vi "create stack file name.vi"(8 "error in (no error)":errorcluster, 10 "name or relative path":string, 11 "Autofocus in":refnum<class "Autofocus.lvclass">) -> (0 "error out":errorcluster, 1 "stack base_xy":path, 3 "Autofocus out":refnum<class "Autofocus.lvclass">)   [LabVIEW 2012, in "Autofocus.lvclass"]
uses:
  Autofocus.lvclass
  Autofocus.lvclass/Autofocus.ctl
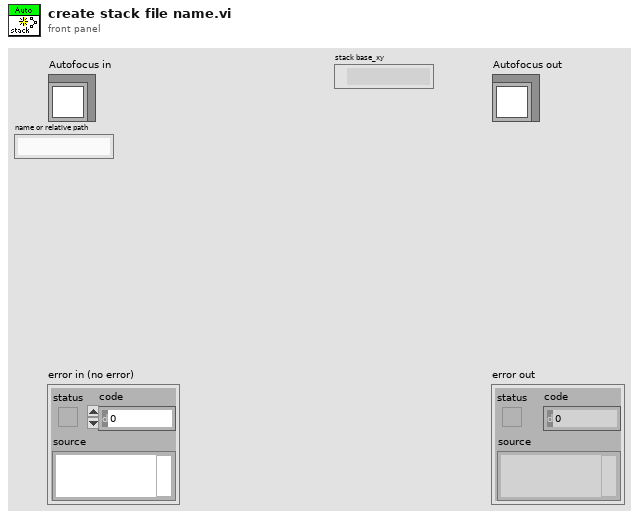
[diagram p1: front panel]
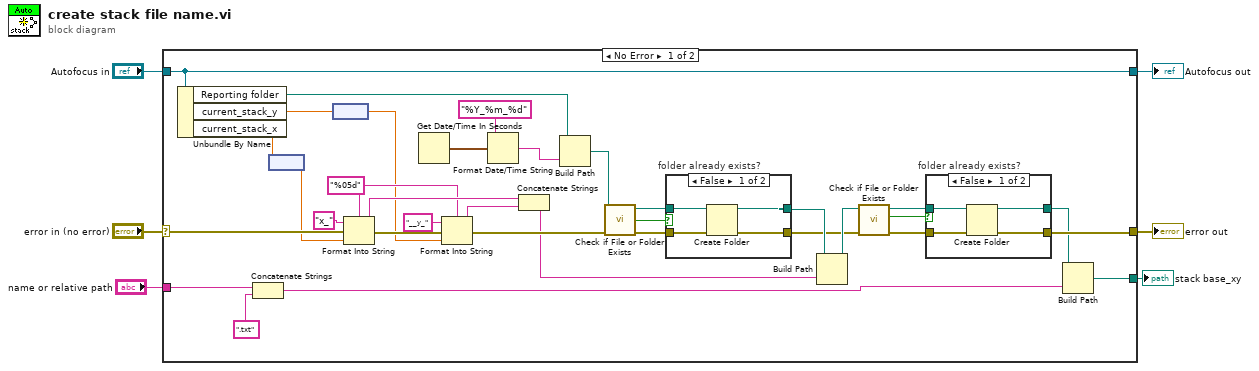
[diagram p0: block diagram]
diagram:
  n1 = case shown="No Error" "error in (no error)" {
    selector: "error in (no error)" -> [w31 w54]
    tunnel: [w15 w54] -> w5
    tunnel: [w40 w53] -> w3
    tunnel: "Autofocus in" -> [w40 w53]
    tunnel: [w19 _] -> w2
    tunnel: "name or relative path" -> [w17 _]
    frame No Error {
      w37 = "%05d" ("format string")
      n2 = Unbundle By Name(w40) -> ("Reporting folder"=w27:path, "current_stack_y"=w32:dbl[unit], "current_stack_x"=w33:dbl[unit])
      n3 = Concatenate Strings(w17, ".txt" ("string")) -> (w16:string)
      n4 = node(w33) -> (w7:dbl)
      n5 = node(w32) -> (w8:dbl)
      n6 = Format Into String(format string=w37, initial string="x_", error in=w31, w7) -> (resulting string=w38:string, error out=w34:errorcluster)
      n7 = Get Date/Time In Seconds() -> (seconds since 1Jan1904=w28:timestamp)
      n8 = Format Into String(format string=w37, initial string="__y_", error in=w34, w8) -> (resulting string=w39:string, error out=w23:errorcluster)
      n9 = Format Date/Time String(time format string (%c)="%Y_%m_%d", seconds (now)=w28) -> (date/time string=w30:string)  [unwired: 1 in]
      n10 = Concatenate Strings(w38, w39) -> (w20:string)
      n11 = Build Path(base path=w27, name or relative path=w30) -> (appended path=w22:path)
      n12 = call <vilib>:"Check if File or Folder Exists.vi"("error in (no error)"=w23, "path"=w22) -> ("error out"=w25:errorcluster, "file or folder exists?"=w24:bool, "dup path"=w26:path)  [unwired: 7 in]
      n13 = case "folder already exists?" shown="False" w24 {
        tunnel: [w48 w52] -> w10
        tunnel: w25 -> [w50 w52]
        tunnel: w26 -> [w49 w51]
        tunnel: [w47 w51] -> w21
        frame False {
          n14 = Create Folder(path (use dialog)=w49, error in=w50) -> (created path=w47:path, error out=w48:errorcluster)  [unwired: 1 in, 1 out]
        }
        frame True {
        }
      }
      n15 = Build Path(base path=w21, name or relative path=w20) -> (appended path=w13:path)
      n16 = call <vilib>:"Check if File or Folder Exists.vi"("error in (no error)"=w10, "path"=w13) -> ("error out"=w11:errorcluster, "file or folder exists?"=w9:bool, "dup path"=w12:path)  [unwired: 7 in]
      n17 = case "folder already exists?" shown="False" w9 {
        tunnel: [w42 w46] -> w15
        tunnel: w11 -> [w44 w46]
        tunnel: w12 -> [w43 w45]
        tunnel: [w41 w45] -> w14
        frame False {
          n18 = Create Folder(path (use dialog)=w43, error in=w44) -> (created path=w41:path, error out=w42:errorcluster)  [unwired: 1 in, 1 out]
        }
        frame True {
        }
      }
      n19 = Build Path(base path=w14, name or relative path=w16) -> (appended path=w19:path)
    }
    frame Error {
    }
  }
  "error out" <- w5
  "Autofocus out" <- w3
  "stack base_xy" <- w2
